vi "TestAdm_ReadSequenceFile.vi"(1 "Path":path, 5 "error in (no error)":errorcluster) -> (14 "Input Buffer":string[](array[string]), 15 "Step paths":string[](array[string]), 16 "Step names":string[](array[string]), 19 "error out":errorcluster)   [LabVIEW 2010]
uses:
  <vilib>/Utility/config.llb/Read Key (String).vi
  <vilib>/Utility/config.llb/NI_LVConfig.lvlib
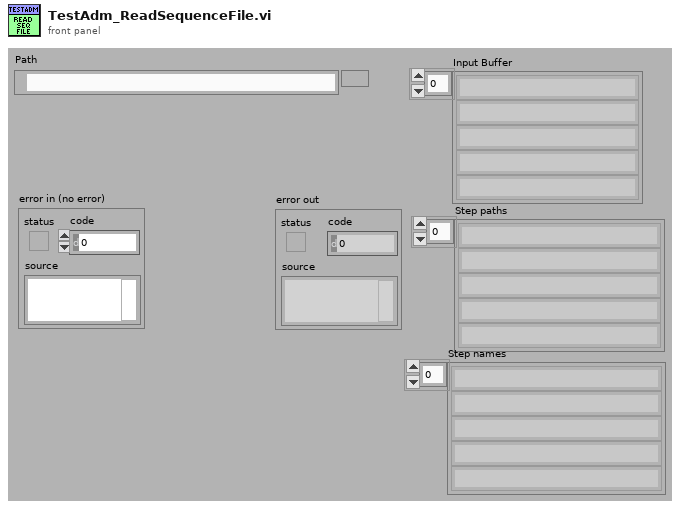
[diagram p1: front panel]
types:
  T1 = typedef "NI_LVConfig.lvlib/Config Data RefNum.ctl" = refnum<k1>
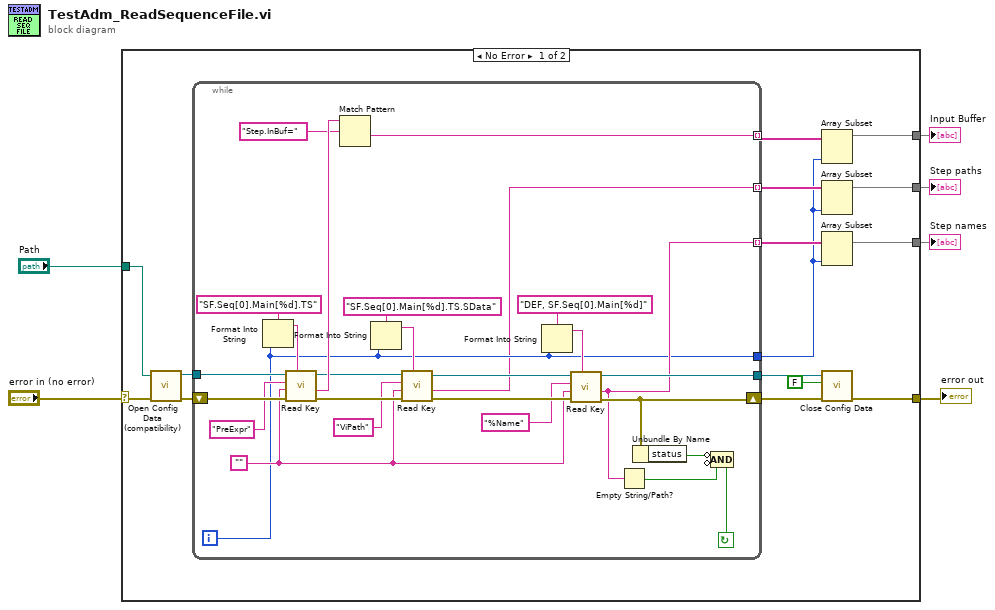
[diagram p0: block diagram]
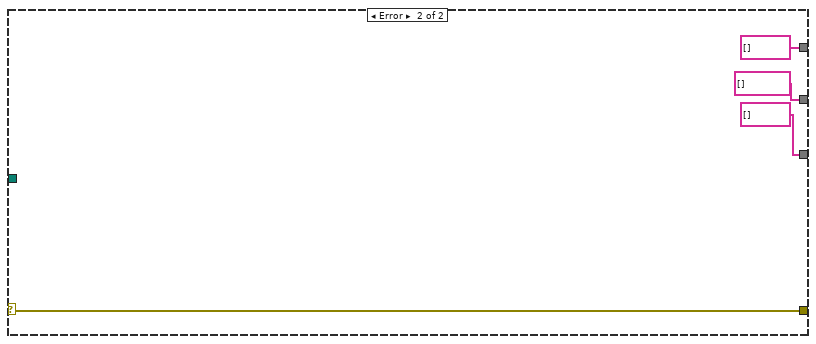
[diagram p2: hidden frame]
diagram:
  n1 = case shown="No Error" "error in (no error)" {
    selector: "error in (no error)" -> [w16 w52]
    tunnel: "Path" -> [w21 _]
    tunnel: [w17 w52] -> w5
    tunnel: [w14 string[] []] -> w3
    tunnel: [w12 string[] []] -> w2
    tunnel: [w10 string[] []] -> w1
    frame No Error {
      n2 = call <vilib>:"Open Config Data (compatibility).vi"("error in (no error)"=w16, "configuration file path"=w21) -> ("error out"=w20:errorcluster, "refnum"=w19:T1)  [unwired: 7 in, 1 out]
      n3 = while {
        tunnel: [w23] -> w9
        tunnel: [w32] -> w18
        tunnel: [w24] -> w11 mode=indexing
        tunnel: [w22] -> w13 mode=indexing
        tunnel: [w42] -> w15 mode=indexing
        tunnel: w19 -> [w47]
        shift-left: w20 -> [w48]
        shift-right: [w33] -> w8
        i -> [w23]
        stop <- w26 continue-if-true
        w28 = ""
        n4 = Format Into String(format string="SF.Seq[0].Main[%d].TS" ("Format String"), w23) -> (resulting string=w45:string)  [unwired: 2 in, 1 out]
        n5 = call-poly <vilib>:"Read Key.vi"("section"=w45, "error in (no error)"=w48, "default value"=w28, "key"="PreExpr", "refnum"=w47) -> ("error out"=w39:errorcluster, "value"=w44:string, "refnum out"=w41:T1)  [unwired: 3 in, 1 out]
        n6 = Match Pattern(string=w44, regular expression="Step.InBuf=") -> (after substring=w42:string)  [unwired: 1 in, 3 out]
        n7 = Format Into String(format string="SF.Seq[0].Main[%d].TS.SData" ("Format String"), w23) -> (resulting string=w38:string)  [unwired: 2 in, 1 out]
        n8 = call-poly <vilib>:"Read Key.vi"("section"=w38, "error in (no error)"=w39, "default value"=w28, "key"="ViPath", "refnum"=w41) -> ("error out"=w37:errorcluster, "value"=w22:string, "refnum out"=w36:T1)  [unwired: 3 in, 1 out]
        n9 = Format Into String(format string="DEF, SF.Seq[0].Main[%d]" ("Format String"), w23) -> (resulting string=w35:string)  [unwired: 2 in, 1 out]
        n10 = call-poly <vilib>:"Read Key.vi"("section"=w35, "error in (no error)"=w37, "default value"=w28, "key"="%Name", "refnum"=w36) -> ("error out"=w33:errorcluster, "value"=w24:string, "refnum out"=w32:T1)  [unwired: 3 in, 1 out]
        n11 = Empty String/Path?(string/path=w24) -> (empty?=w25:bool)
        n12 = Unbundle By Name(w33) -> ("status"=w27:bool)
        n13 = Compound Arithmetic op=AND(invert w27, invert w25) -> (w26:bool)
      }
      n14 = Array Subset(array=w15, length=w9) -> (w14:string[])  [unwired: 1 in]
      n15 = Array Subset(array=w13, length=w9) -> (w12:string[])  [unwired: 1 in]
      n16 = Array Subset(array=w11, length=w9) -> (w10:string[])  [unwired: 1 in]
      n17 = call <vilib>:"Close Config Data.vi"("error in (no error)"=w8, "write file if changed (T)"=FALSE ("write configuration file? (T)"), "refnum"=w18) -> ("error out"=w17:errorcluster)  [unwired: 7 in, 1 out]
    }
    frame Error {
    }
  }
  "error out" <- w5
  "Input Buffer" <- w3
  "Step paths" <- w2
  "Step names" <- w1
